vi "TERNARY OPERATOR.vi"() -> ()   [LabVIEW 2019]
panel:
  in  "INPUT 2":dbl
  in  "INPUT 1":dbl
  out "OUTPUT":string
  # "TERNARY OPERATOR"
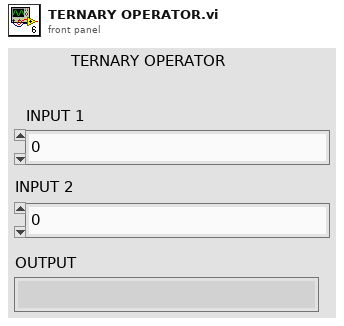
[diagram p1: front panel]
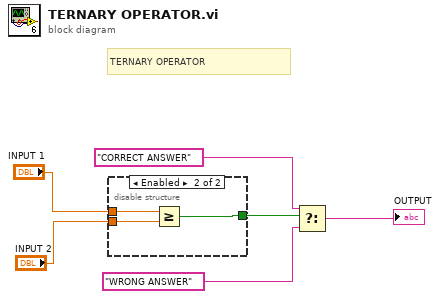
[diagram p0: block diagram]
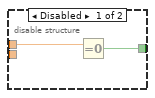
[diagram p2: hidden frame]
diagram:
  # "TERNARY OPERATOR"
  n1 = disable-structure shown="Enabled" {
    disable-tunnel: [w8 w11] -> w6
    disable-tunnel: "INPUT 1" -> [w7 w10]
    disable-tunnel: "INPUT 2" -> [_ w9]
    frame Disabled {
      n2 = Equal To 0?(x=w7) -> (x = 0?=w8:bool)
    }
    frame Enabled {
      n3 = Greater Or Equal?(x=w10, y=w9) -> (x >= y?=w11:bool)
    }
  }
  n4 = Select(t="CORRECT ANSWER", s=w6, f="WRONG ANSWER") -> (s? t:f=→"OUTPUT":string)
